vi "belt safety.vi"(1 "Input":dbl) -> (0 "Safe Output":dbl)   [LabVIEW 2013]
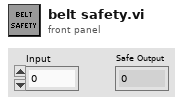
[diagram p1: front panel]
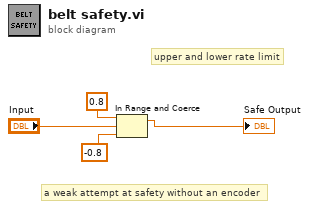
[diagram p0: block diagram]
diagram:
  # "a weak attempt at safety without an encoder"
  # "upper and lower rate limit"
  n1 = In Range and Coerce(upper limit=0.8, x="Input", lower limit=-0.8 ("upper limit")) -> (coerced(x)=→"Safe Output":dbl)  [unwired: 1 out]
